vi "DAQmx Create Channel (AI-Voltage-RMS).vi"(0 "task in":refnum<k21>, 1 "maximum value":dbl=5.0 format="%0.2f", 2 "minimum value":dbl=-5.0 format="%0.2f", 3 "input terminal configuration":i32(ring)=-1 items=["Default"=-1, "RSE"=10083, "NRSE"=10078, "Differential"=10106, "Pseudodifferential"=12529], 5 "physical channels":tag, 7 "name to assign":string, 9 "units":i32(ring)=10348 items=["Volts"=10348, "From Custom Scale"=10065], 11 "error in":errorcluster, 12 "custom scale name":tag) -> (4 "task out":refnum<k21>, 15 "error out":errorcluster)   [LabVIEW 2013]
doc: "Creates channel(s) to measure voltage RMS, the average (mean) power of the acquired voltage."
uses:
  nilvaiu.dll
panel:
  # "input limits"
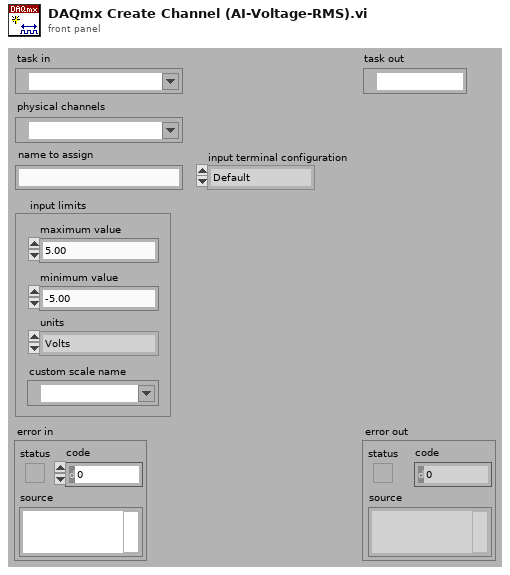
[diagram p1: front panel]
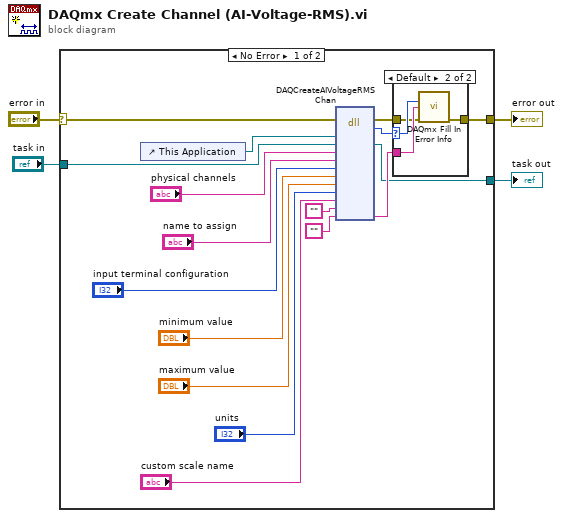
[diagram p0: block diagram]
diagram:
  n1 = case shown="No Error" "error in" {
    selector: "error in" -> [w8 w27]
    tunnel: "task in" -> [w10 w28]
    tunnel: [w7 w28] -> w3
    tunnel: [w9 w27] -> w2
    frame No Error {
      n2 = control-ref of="This Application"() -> (w11:refnum<vi>)
      n3 = dll-call lib="nilvaiu.*" fn="DAQCreateAIVoltageRMSChan"(error in=w8, "lvAppRef"=w11, "refObjPtr"=w10, "physicalChannelName"="physical channels", "channelNameIn"="name to assign", "terminalConfig"="input terminal configuration", "minVal"="minimum value", "maxVal"="maximum value", "units"="units", "customScaleName"="custom scale name", "channelNamesOut"="", "extendedErrorInfo"="") -> (error out=w21:errorcluster, "return type"=w20:i32, "refObjPtr"=w7:refnum<k21>, "extendedErrorInfo"=w19:string)  [unwired: 11 in, 1 out]
      n4 = case shown="Default" w20 {
        selector: w20 -> [_ w25]
        tunnel: w21 -> [w22 w23]
        tunnel: [w22 w26] -> w9
        tunnel: w19 -> [_ w24]
        frame 0 {
        }
        frame Default {
          n5 = call "DAQmx Fill In Error Info.vi"("status code"=w25, "extended error info"=w24, "error in"=w23) -> ("error out"=w26:errorcluster)  [unwired: 1 in, 11 out]
        }
      }
    }
    frame Error {
    }
  }
  "task out" <- w3
  "error out" <- w2
